vi "Test Get Table Values (VAR).vi"(11 "Test Case In":refnum<class "Test Open Xml.lvclass">) -> (0 "error out":errorcluster, 3 "Test Case Out":refnum<class "Test Open Xml.lvclass">)   [LabVIEW 2020, in "Test Open Xml.lvclass"]
uses:
  Test Open Xml.lvclass
  Source/Open Xml.lvlib
  0a0d70f3-36fe-46ba-8b3e-e6c07e708d9f.vi
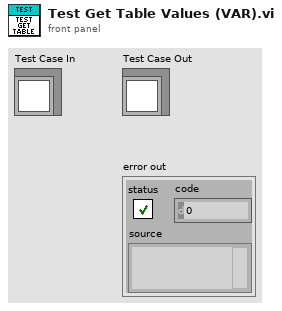
[diagram p1: front panel]
types:
  T1 = cluster{"Sheet Name":string, "Name":string, "Display Name":string, "Range":string}
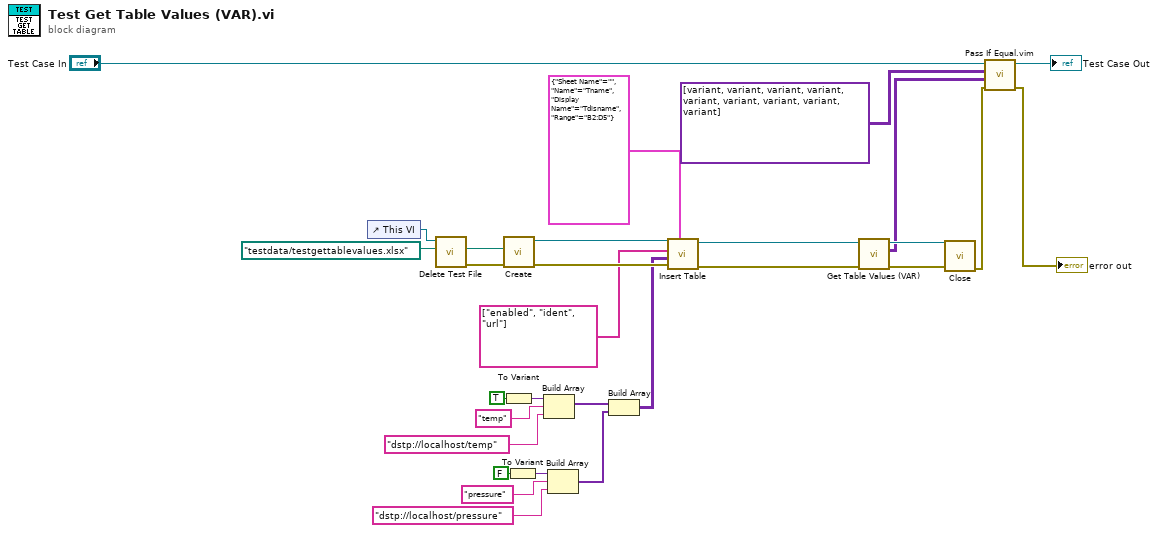
[diagram p0: block diagram]
diagram:
  n1 = control-ref of="This VI"() -> (w21:refnum<vi>)
  n2 = call "Delete Test File.vi"("name or relative path"=path "testdata/testgettablevalues.xlsx", "VI in"=w21) -> ("error out"=w22:errorcluster, "deleted path"=w23:path)  [unwired: 8 in]
  n3 = call "Create.vi"("error in"=w22, "Path"=w23) -> ("error out"=w18:errorcluster, "SpreadsheetDoc"=w19:refnum<k24>)  [unwired: 8 in]
  n4 = To Variant(anything=TRUE) -> (Variant=w15:variant)
  n5 = To Variant(anything=FALSE) -> (Variant=w10:variant)
  n6 = Build Array(w15, "temp", "dstp://localhost/temp") -> (w8:variant[])
  n7 = Build Array(w10, "pressure", "dstp://localhost/pressure") -> (w7:variant[])
  n8 = Build Array(w8, w7) -> (w3:variant[][])
  n9 = call "Insert Table.vi"("Location"=T1 {"Sheet Name"="", "Name"="Tname", "Display Name"="Tdisname", "Range"="B2:D5"}, "error in"=w18, "Cell Values"=w3, "Header Names"=string[] ["enabled", "ident", "url"], "SpreadsheetDoc in"=w19) -> ("error out"=w25:errorcluster, "SpreadsheetDoc out"=w5:refnum<k24>)  [unwired: 5 in]
  n10 = call "Get Table Values (VAR).vi"("error in"=w25, "SpreadsheetDoc in"=w5) -> ("error out"=w6:errorcluster, "Table Values"=w2:variant[][], "SpreadsheetDoc out"=w4:refnum<k24>)  [unwired: 7 in]
  n11 = call "Close.vi"("error in"=w6, "SpreadsheetDoc"=w4) -> ("error out"=w26:errorcluster)  [unwired: 9 in]
  n12 = call "Pass If Equal.vim"("error in (no error)"=w26, "Actual"=w2, "Expected"=variant[][] [[variant(bool TRUE), variant(string "temp"), variant(string "dstp://localhost/temp")], [variant(bool FALSE), variant(string "pressure"), variant(string "dstp://localhost/pressure")], [variant, variant, variant]] ("Cell Values"), "LUnit Test Case In"="Test Case In") -> ("error out"=→"error out":errorcluster, "LUnit Test Case Out"=→"Test Case Out":refnum<class "Test Open Xml.lvclass">)  [unwired: 6 in]
